vi "Hindbrain Main.vi"(8 "Boat Type":T1, 9 "XBee Serial Port":refnum<visa-resource-name>="LPT1", 11 "NotifierReff":T5) -> ()   [LabVIEW 2013]
doc: "Place to hold all the hindbrain code."
uses:
  Data/TypeDefs/Notifiers.ctl
  Data/TypeDefs/UTM Location.ctl
  Data/TypeDefs/Sail Set Suggestions.ctl
  Data/TypeDefs/Rudder Set Suggestions.ctl
  Data/TypeDefs/OverrideInformation.ctl
  Data/TypeDefs/OverrideMode.ctl
  Data/TypeDefs/MotorSetup.ctl
  Data/TypeDefs/DynamixelSetupInfo.ctl
  Data/TypeDefs/AirmarStatus.ctl
  Data/TypeDefs/HardwareOnline.ctl
  Data/TypeDefs/DynamixelCycleTracker.ctl
  Data/TypeDefs/RC Input Values.ctl
  Classes/Waypoint/Waypoint.lvclass
  Data/TypeDefs/BoatType.ctl
  <vilib>/myRIO/Common/Instrument Driver Framework/myRIO v1.0/UART/vis/myRIO v1.0 Close UART.vi
  <vilib>/myRIO/Common/Instrument Driver Framework/Utilities/vis/FPGA Ref Manager.vi
  <vilib>/myRIO/Common/Instrument Driver Framework/myRIO v1.0/myRIO v1.0 Reset FPGA.vi
  <vilib>/myRIO/Instrument Drivers/Utilities/Utilities.lvlib
  <instrlib>/Dynamixel Motor/Dynamixel Motor.lvlib
panel:
  in  "Tab Control":T2(tab)
  out "Write loop\ncounter":i32
  out "Commanded rudder value":T3 min=-0.95 max=0.95 scale=1.0..-1.0
  out "Commanded sail value":dbl
  out "Dynamixel\nPositions (deg)":dbl[](array[numeric])
  in  "Read actions per\nwrite action":i32=4
  out "Think Counter":i32
  out "Think Heartbeat":bool
  out "Sense Counter":i32
  out "Sense Heartbeat":bool
  out "Act Heartbeat":bool
  out "Read loop counter":i32
  out "Updated Dynamixel Cycles":T4
  in  "Motors Enabled":bool[](array[boolean])=[TRUE, TRUE, TRUE]
  out "Hemisphere Counter":i32
  out "Airmar Counter":i32
  out "Hemi Compass":dbl
  out "Airmar Compass":dbl
  out "String written to XBee":string
  out "String received from XBee":string
  out "UDP Time Out?":bool
  out "Battery Volts":dbl
  out "Replace? (<6?)":bool
  in  "Wind Speed":dbl
  out "XBee Sense/Act Counter":i32
  out "XBee Sense/Act Heartbeat":bool
  out "Camera Sense Counter":i32
  out "Camera Sense Heartbeat":bool
  out "Think Counter":i32
  out "Think Heartbeat":bool
  # "Timing"
  # "Timing"
  # "If you're getting no strings, do you have the right COM port?"
  # "Camera"
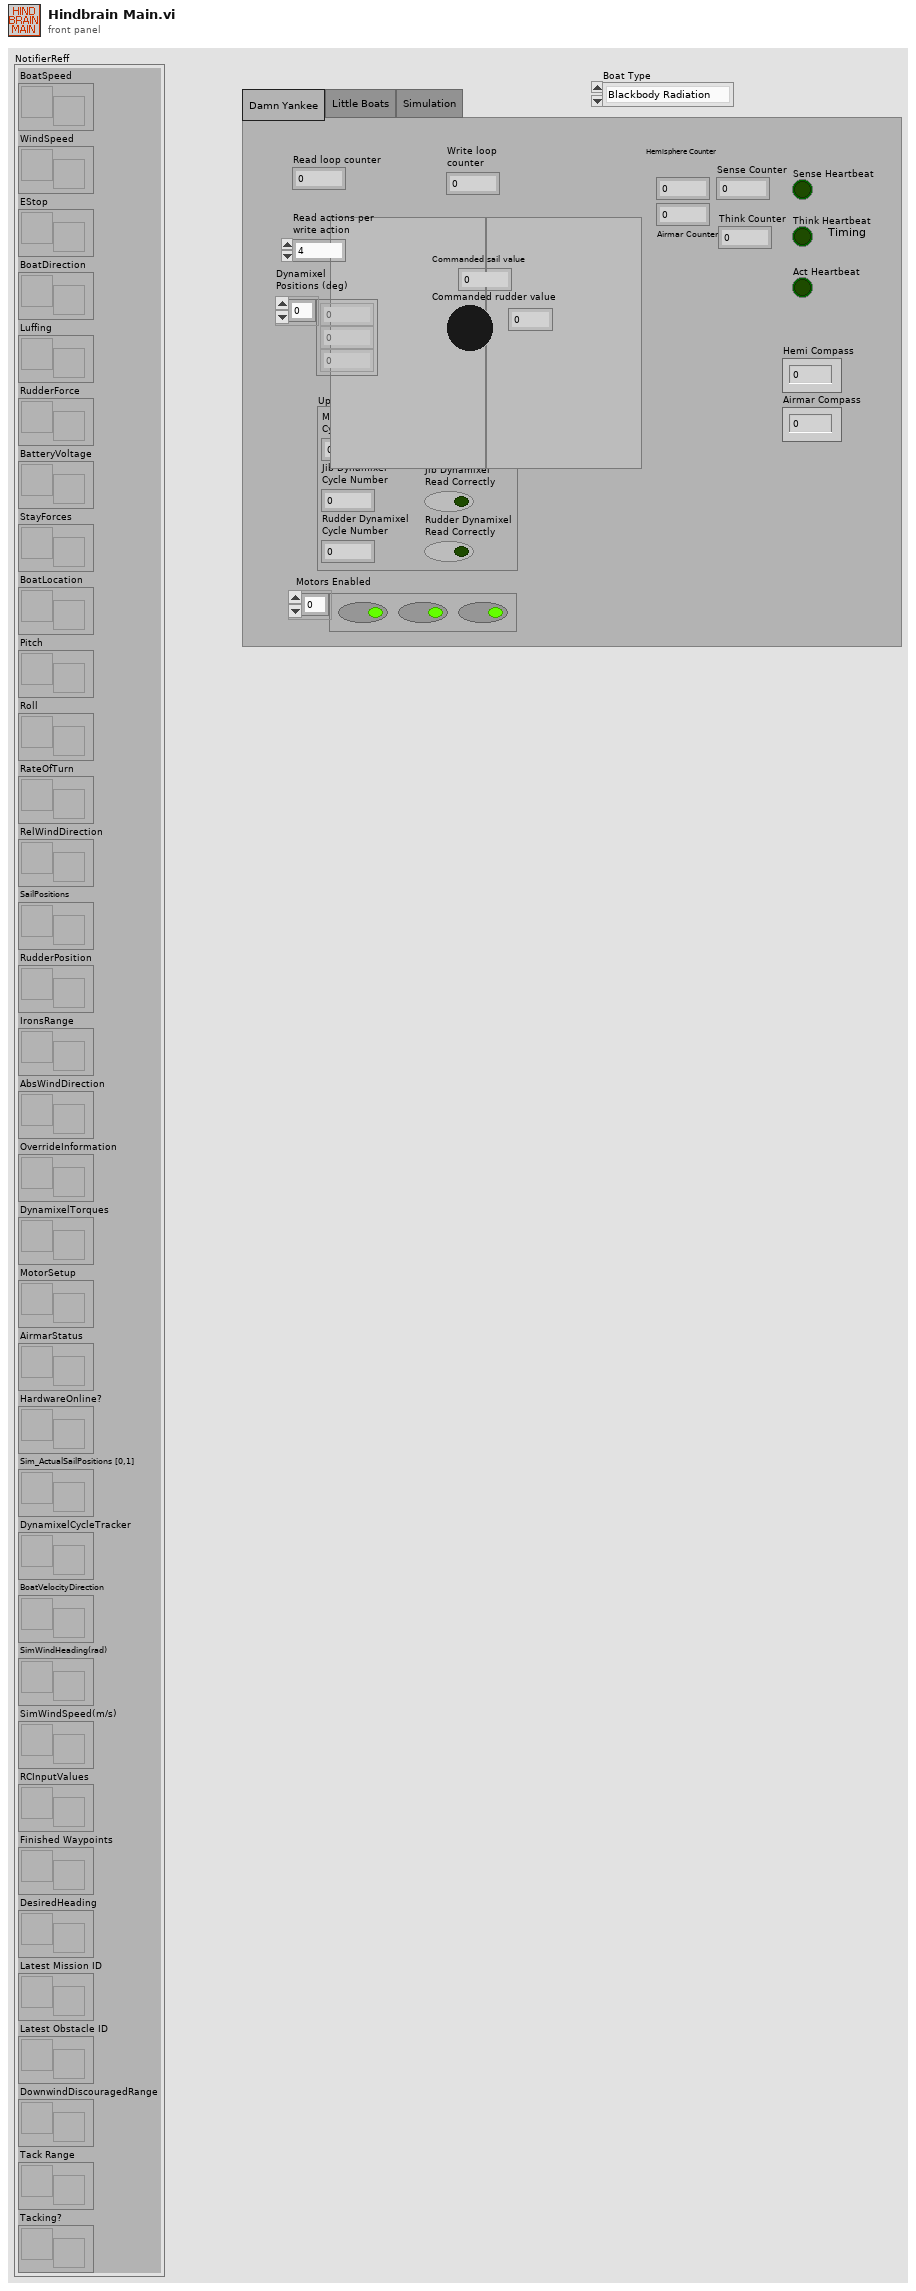
[diagram p1: front panel]
types:
  T1 = typedef "BoatType.ctl" = enum16{"Blackbody Radiation", "ReadLog", "Little boats", "Damn Yankee"}
  T2 = enum32{"Damn Yankee", "Little Boats", "Simulation"}
  T3 = typedef "Rudder Set Suggestions.ctl" = dbl
  T4 = typedef "DynamixelCycleTracker.ctl" = cluster{"Main Dynamixel\nCycle Number":i32, "Jib Dynamixel\nCycle Number":i32, "Rudder Dynamixel\nCycle Number":i32, "Main Dynamixel\nRead Correctly":bool, "Jib Dynamixel\nRead Correctly":bool, "Rudder Dynamixel\nRead Correctly":bool}
  T5 = typedef "Notifiers.ctl" = cluster{"BoatSpeed":refnum<notifier>, "WindSpeed":refnum<notifier>, "EStop":refnum<notifier>, "BoatDirection":refnum<notifier>, "Luffing":refnum<notifier>, "RudderForce":refnum<notifier>, "BatteryVoltage":refnum<notifier>, "StayForces":refnum<notifier>, "BoatLocation":refnum<notifier>, "Pitch":refnum<notifier>, "Roll":refnum<notifier>, "RateOfTurn":refnum<notifier>, "RelWindDirection":refnum<notifier>, "SailPositions":refnum<notifier>, "RudderPosition":refnum<notifier>, "IronsRange":refnum<notifier>, "AbsWindDirection":refnum<notifier>, "OverrideInformation":refnum<notifier>, "DynamixelTorques":refnum<notifier>, "MotorSetup":refnum<notifier>, "AirmarStatus":refnum<notifier>, "HardwareOnline?":refnum<notifier>, "Sim_ActualSailPositions [0,1]":refnum<notifier>, "DynamixelCycleTracker":refnum<notifier>, "BoatVelocityDirection":refnum<notifier>, "SimWindHeading(rad)":refnum<notifier>, "SimWindSpeed(m/s)":refnum<notifier>, "RCInputValues":refnum<notifier>, "Finished Waypoints":refnum<notifier>, "DesiredHeading":refnum<notifier>, "Latest Mission ID":refnum<notifier>, "Latest Obstacle ID":refnum<notifier>, "DownwindDiscouragedRange":refnum<notifier>, "Tack Range":refnum<notifier>, "Tacking?":refnum<notifier>}
  T6 = typedef "GPS-Compass Queue Cluster.ctl" = cluster{"BoatLocation Queue":refnum<queue>, "BoatDirection Queue":refnum<queue>, "BoatSpeed Queue":refnum<queue>, "RateOfTurn Queue":refnum<queue>, "Pitch Queue":refnum<queue>, "Roll Queue":refnum<queue>, "BoatVelocityDirection Queue ":refnum<queue>}
  T7 = typedef "WindData Queue Cluster.ctl" = cluster{"RelWindDirection Queue":refnum<queue>, "WindSpeed Queue":refnum<queue>, "AbsWindDirection Queue":refnum<queue>}
  T8 = cluster{"Shroud Queue":refnum<queue>, "Battery Voltage Queue":refnum<queue>, "Accelerometer Queue":refnum<queue>, "AirmarGPS-Compass Queue Cluster":T6, "Hemisphere Queue Cluster":T6, "Airmar Wind Queue Cluster":T7, "Wind Vane Queue Cluster":T7, "Little Boat Queues":cluster{"Heading Queue":refnum<queue>, "Location Queue":refnum<queue>, "Wind Speed Queue":refnum<queue>, "Tilt Queue":refnum<queue>, "Wind Direction Queue":refnum<queue>}, "DynamixelTorque Queue":refnum<queue>, "DynamixelPosition Queue":refnum<queue>}
  T9 = typedef "MotorSetup.ctl" = cluster{"Main Dynamixel Set Data":T10, "Rudder Dynamixel Set Data":T10, "Jib Dynamixel Set Data":T10}
  T10 = typedef "DynamixelSetupInfo.ctl" = cluster{"Lower Winch Bound (deg)":dbl, "Upper Winch Bound (deg)":dbl}
  T11 = typedef "DamnYankeeIOPorts.ctl" = cluster{"Airmar VISA Resource":refnum<visa-resource-name>, "Hemisphere VISA Resource":refnum<visa-resource-name>, "Dynamixel VISA Resource":refnum<visa-resource-name>, "Airmar Error":errorcluster, "Hemisphere Error":errorcluster, "Dynamixel Error":errorcluster, "FPGA Error":errorcluster, "FPGA VI Reference Out":refnum<k20>, "Motors IDs Found":u8[]}
  T12 = cluster{"Heading Queue":refnum<queue>, "Location Queue":refnum<queue>, "Wind Speed Queue":refnum<queue>, "Tilt Queue":refnum<queue>, "Wind Direction Queue":refnum<queue>}
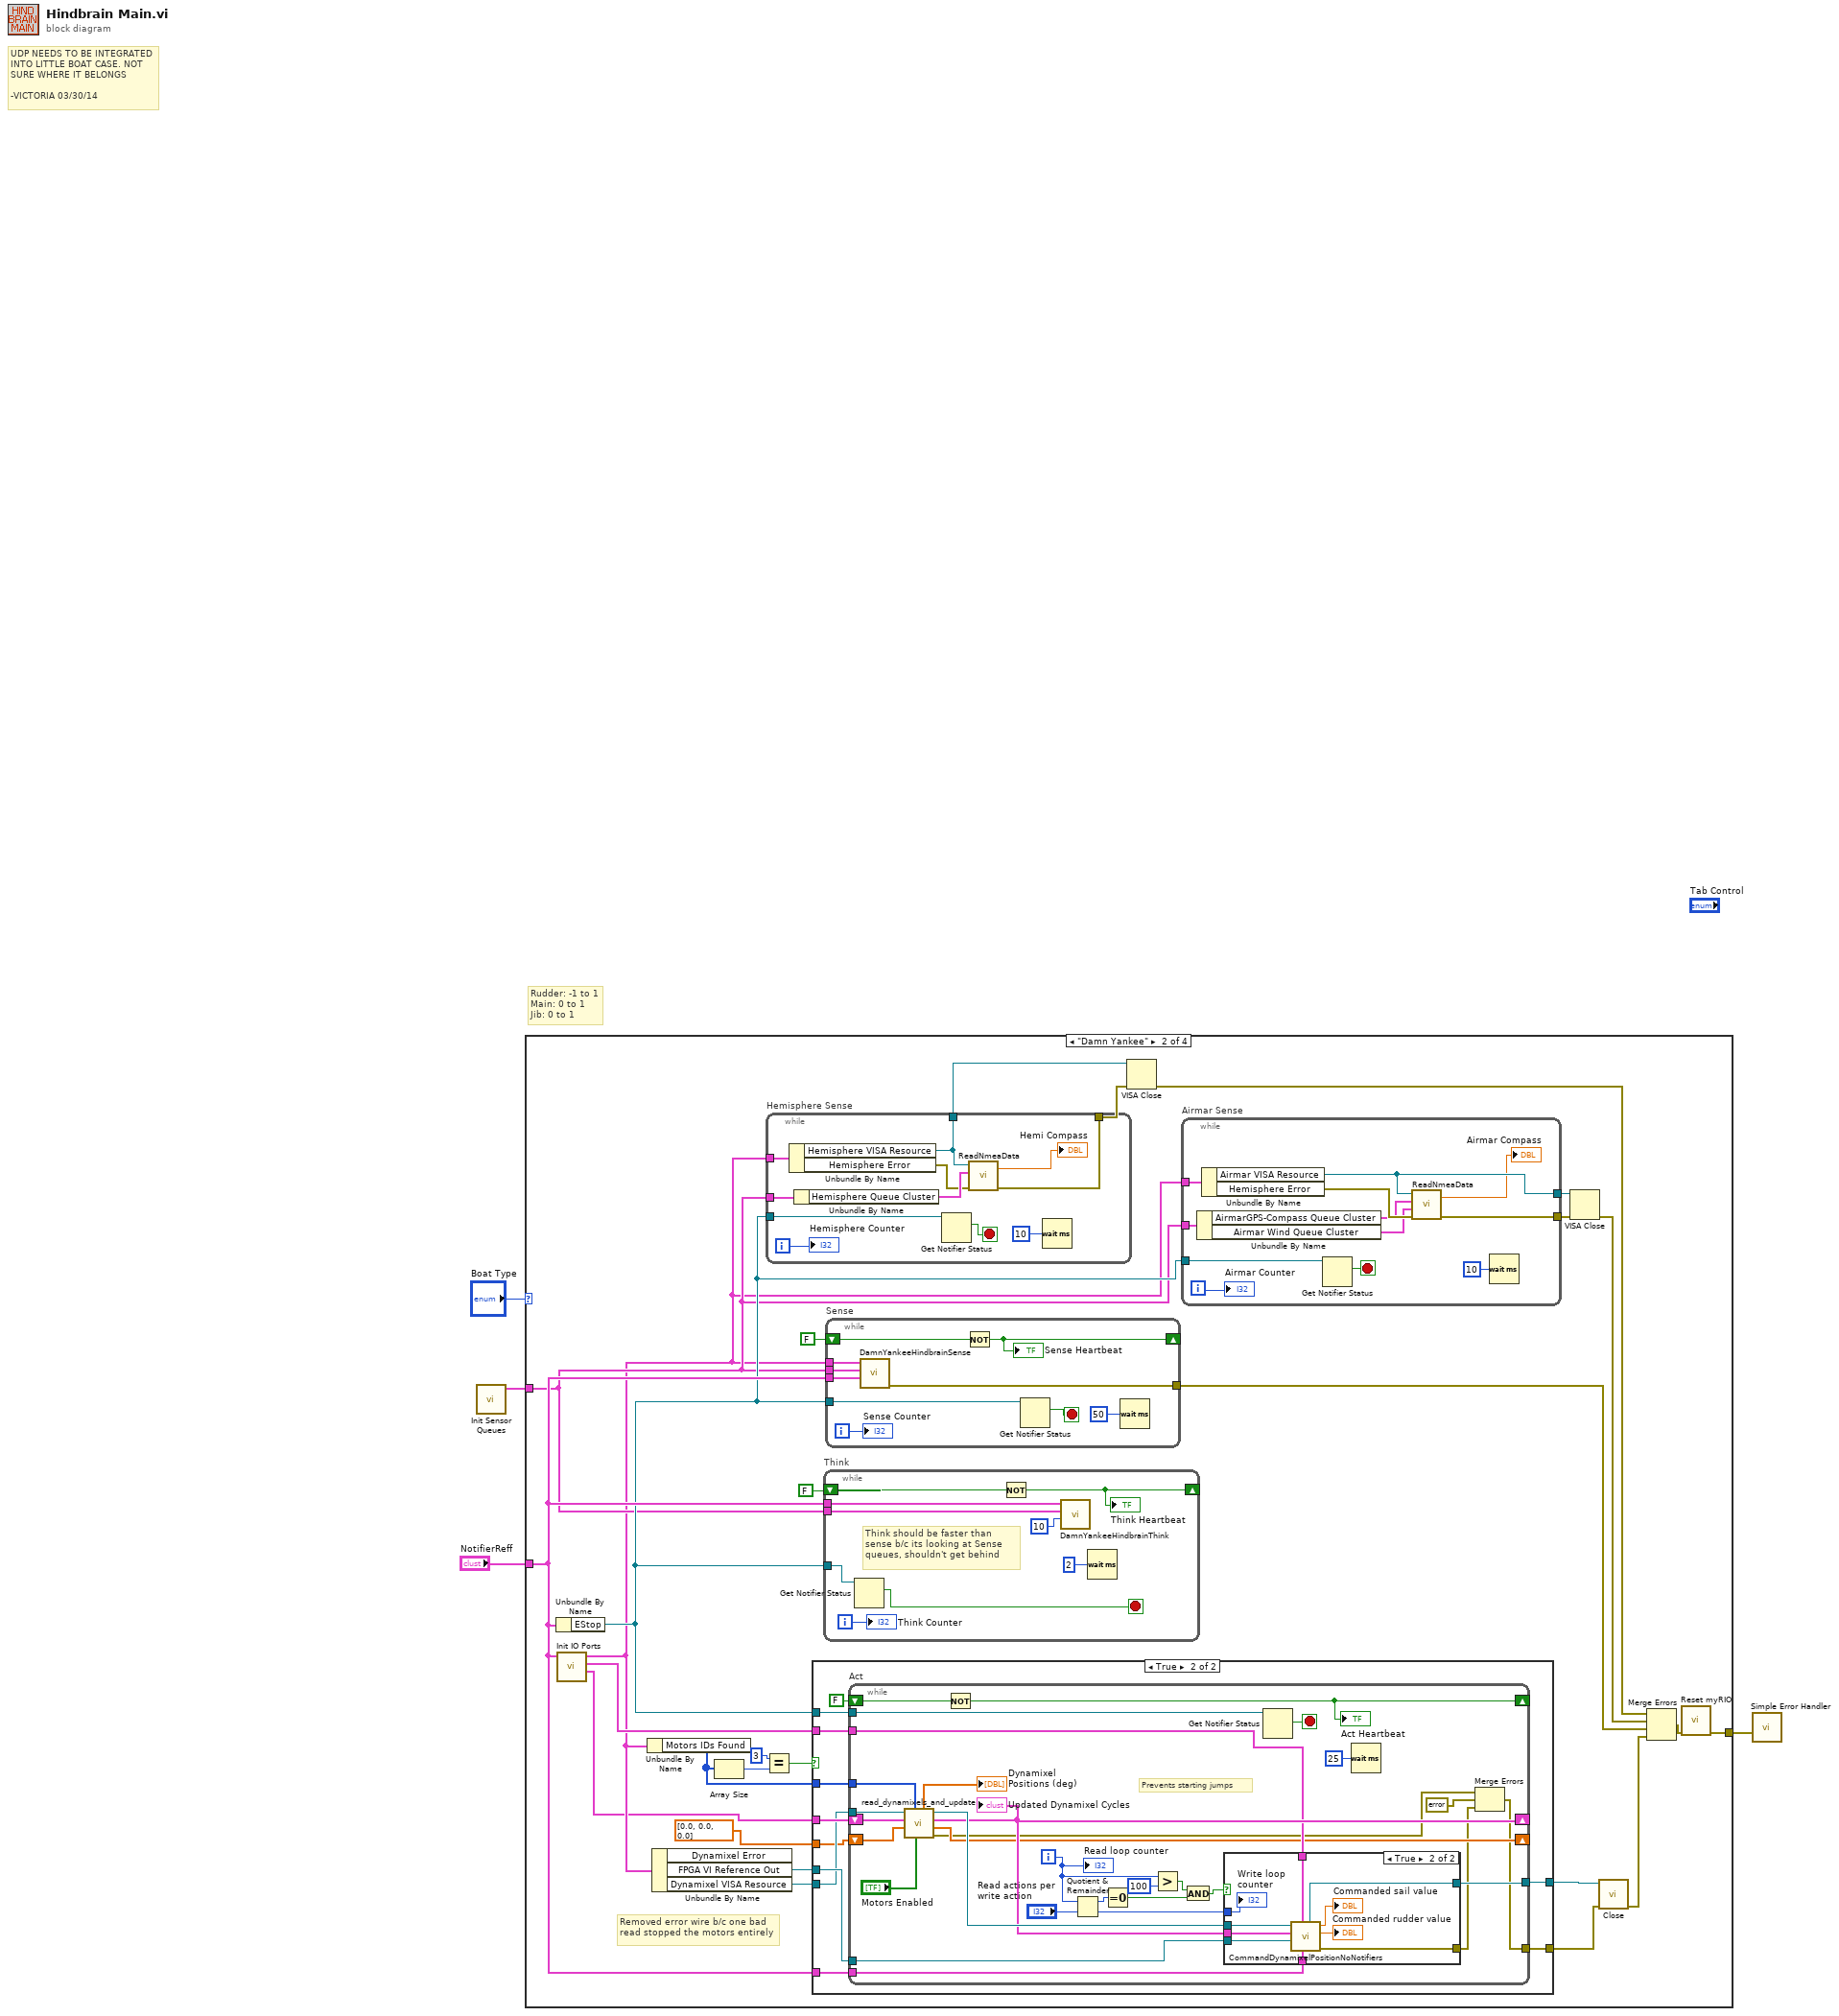
[diagram p0: block diagram]
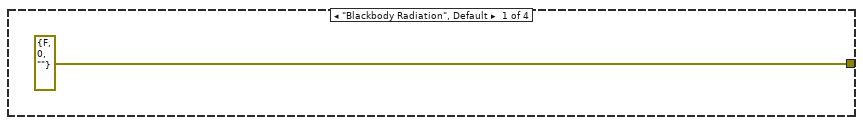
[diagram p2: hidden frame]
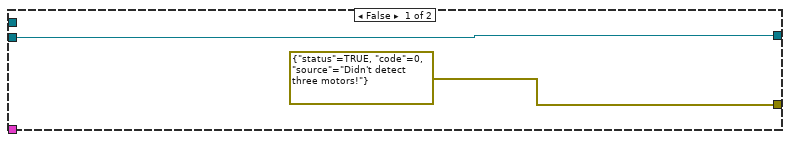
[diagram p3: hidden frame]
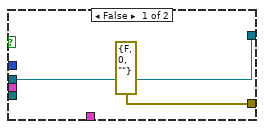
[diagram p4: hidden frame]
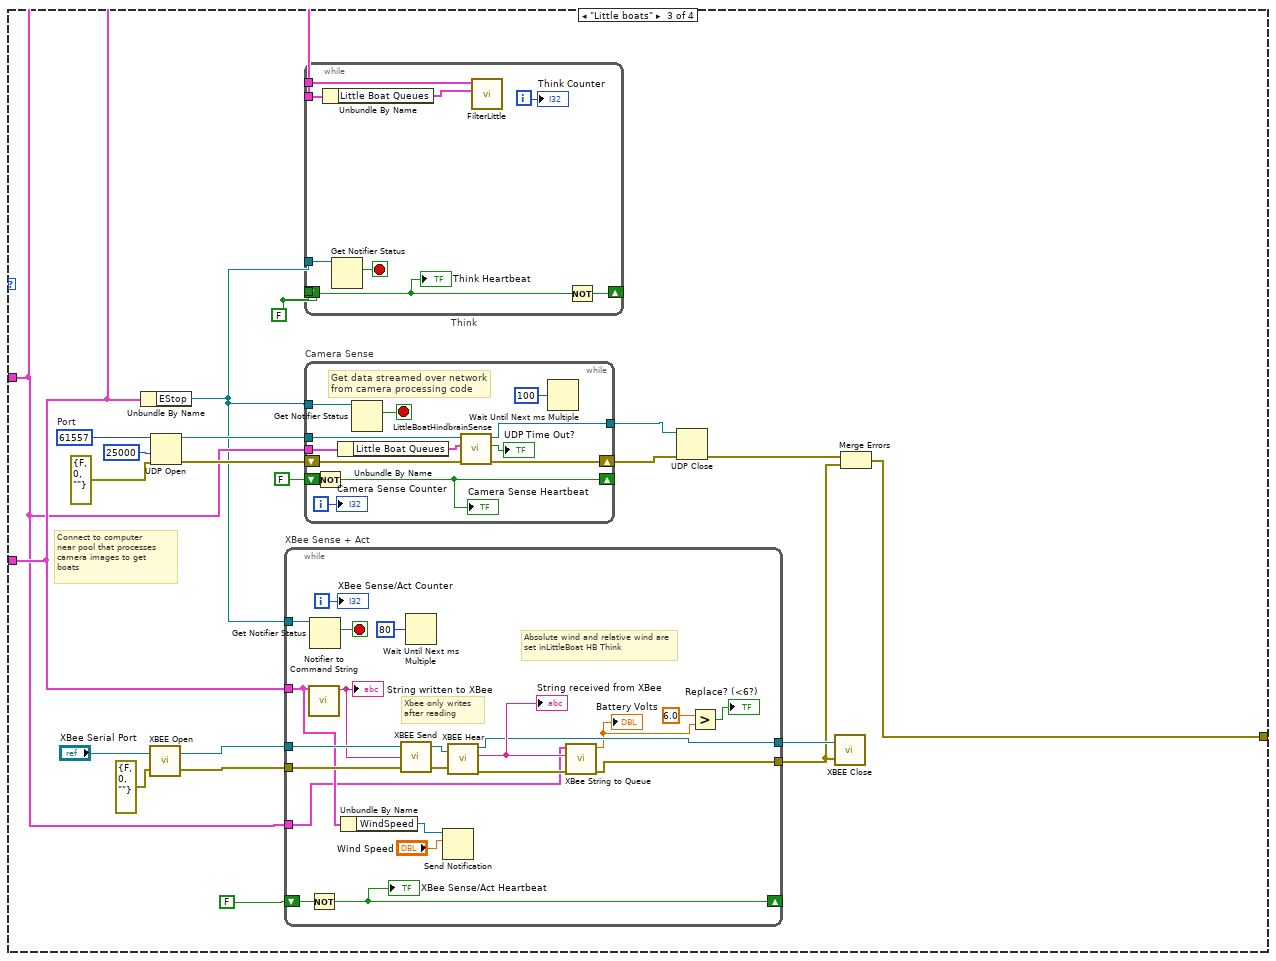
[diagram p5: hidden frame]
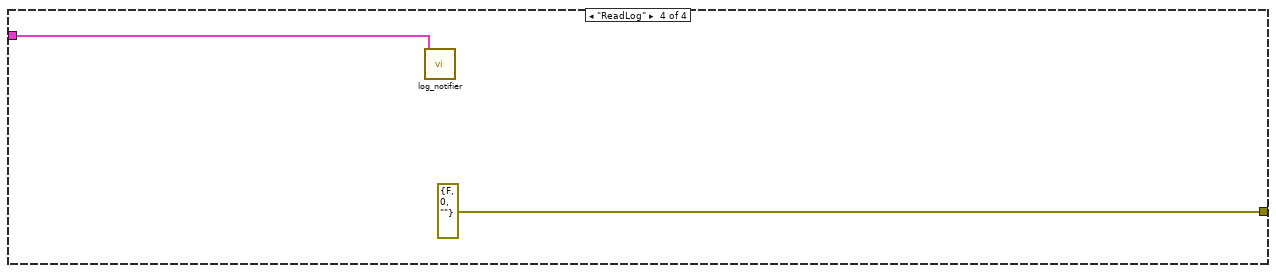
[diagram p6: hidden frame]
diagram:
  # "Rudder: -1 to 1\nMain: 0 to 1 \nJib: 0 to 1"
  # "UDP NEEDS TO BE INTEGRATED\nINTO LITTLE BOAT CASE. NOT \nSURE WHERE IT BELONGS\n\n-VICTORIA 03/30/14"
  n1 = call "Init Sensor Queues.vi"() -> ("output cluster"=w4:T8)  [unwired: 11 in]
  n2 = case shown="\"Damn Yankee\"" "Boat Type" {
    tunnel: w4 -> [_ w15 w139 _]
    tunnel: "NotifierReff" -> [_ w18 w143 w194]
    tunnel: [errorcluster {"status"=FALSE, "code"=0, "source"=""} ("error IO") w31 w150 errorcluster {"status"=FALSE, "code"=0, "source"=""} ("error IO")] -> w3
    frame "Blackbody Radiation", Default {
    }
    frame "Damn Yankee" {
      # "Removed error wire b/c one bad read stopped the motors entirely"
      n3 = Unbundle By Name(w18) -> ("EStop"=w16:refnum<notifier>)
      n4 = call "Init IO Ports.vi"("NotifierReff"=w18) -> ("Dynamixel Cycles"=w6:T4, "Dynamixel Bounds Out"=w23:T9, "IO Port Cluster"=w14:T11)  [unwired: 8 in]
      n5 = Unbundle By Name(w14) -> ("Motors IDs Found"=w24:u8[])
      n6 = Unbundle By Name(w14) -> ("FPGA VI Reference Out"=w25:refnum<k20>, "Dynamixel VISA Resource"=w22:refnum<visa-resource-name>)  [unwired: 1 out]
      n7 = Array Size(array=w24) -> (size(s)=w28:i32)
      n8 = Equal?(x=3, y=w28) -> (x = y?=w27:bool)
      n9 = while "Hemisphere Sense" {
        tunnel: w14 -> [w55]
        tunnel: w15 -> [w54]
        tunnel: w16 -> [w50]
        tunnel: [w48] -> w13
        tunnel: [w47] -> w12
        i -> [w51]
        stop <- w49 stop-if-true
        n10 = Unbundle By Name(w55) -> ("Hemisphere VISA Resource"=w48:refnum<visa-resource-name>, "Hemisphere Error"=w52:errorcluster)
        n11 = Unbundle By Name(w54) -> ("Hemisphere Queue Cluster"=w53:T6)
        n12 = Get Notifier Status(notifier=w50) -> (current notification=w49:bool)  [unwired: 1 in, 4 out]
        n13 = call "ReadNmeaData.vi"("error in"=w52, "GPS-Compass Queue Cluster"=w53, "Serial Port"=w48) -> ("error out"=w47:errorcluster, "Boat Direction 2"=→"Hemi Compass":dbl)  [unwired: 2 in, 5 out]
        n14 = Wait (ms)(milliseconds to wait=u32 10) -> ()  [unwired: 1 out]
        "Hemisphere Counter" <- w51
      }
      n15 = case shown="True" w27 {
        tunnel: [errorcluster {"status"=TRUE, "code"=0, "source"="Didn't detect three motors!"} ("error out") w58] -> w20
        tunnel: w16 -> [_ w67]
        tunnel: w23 -> [_ w66]
        tunnel: w6 -> [_ w65]
        tunnel: [w56 w64] -> w21
        tunnel: w25 -> [_ w63]
        tunnel: w24 -> [_ w62]
        tunnel: w22 -> [w56 w61]
        tunnel: w18 -> [_ w60]
        tunnel: dbl[] [0.0, 0.0, 0.0] -> [_ w59]
        frame False {
        }
        frame True {
          n16 = while "Act" {
            tunnel: w66 -> [w85]
            tunnel: w67 -> [w97]
            shift-right: [w96] -> _
            shift-left: FALSE -> [w95]
            shift-right: [w86] -> _
            shift-left: w65 -> [w87]
            tunnel: [w84] -> w64
            shift-right: [w83] -> _
            shift-left: w59 -> [w82]
            tunnel: w63 -> [w79]
            tunnel: w62 -> [w78]
            tunnel: w61 -> [w77]
            tunnel: w60 -> [w76]
            tunnel: [w74] -> w58
            i -> [w71]
            stop <- w98 stop-if-true
            # "Prevents starting jumps"
            n17 = call "read_dynamixels_and_update.vi"("Motors Enabled"="Motors Enabled", "Motors IDs Found"=w78, "Last read positions"=w82, "Dynamixel Cycle Constant"=w87, "VISA Refnum in"=w77) -> ("error out"=w81:errorcluster[], "Latest read positions (dyn)"=w83:dbl[], "Updated Dynamixle Cycles"=w86:T4, "VISA Refnum out"=w92:refnum<visa-resource-name>, "Dynamixel\nPositions (deg)"=→"Dynamixel\nPositions (deg)":dbl[])  [unwired: 2 in]
            "Updated Dynamixel Cycles" <- w86
            n18 = Not(x=w95) -> (.not. x?=w96:bool)
            "Act Heartbeat" <- w96
            n19 = Quotient & Remainder(x=w71, y="Read actions per\nwrite action") -> (x-y*floor(x/y)=w90:i32, floor(x/y)=w89:i32)
            n20 = Equal To 0?(x=w90) -> (x = 0?=w72:bool)
            n21 = Greater?(x=w71, y=100) -> (0:w70:bool)
            n22 = And(x=w70, y=w72) -> (x .and. y?=w73:bool)
            n23 = case shown="True" w73 {
              tunnel: w79 -> [_ w110]
              tunnel: w85 -> [_ w102]
              tunnel: w92 -> [w100 w109]
              tunnel: w86 -> [_ w108]
              tunnel: [errorcluster {"status"=FALSE, "code"=0, "source"=""} ("Error out") w105] -> w75
              tunnel: [w100 w104] -> w84
              tunnel: w89 -> [_ w103]
              tunnel: w76 -> [_ w101]
              frame False {
              }
              frame True {
                n24 = call "CommandDynamixelPositionNoNotifiers.vi"("NotifierReff"=w101, "Dynamixel Bounds"=w102, "FPGA VI Reference In"=w110, "Dynamixel Cycles"=w108, "VISA resource name"=w109) -> ("Error out"=w105:errorcluster, "Commanded rudder value"=→"Commanded rudder value":T3, "Debug sail value"=→"Commanded sail value":dbl, "VISA resource name OUT"=w104:refnum<visa-resource-name>)  [unwired: 3 in]
                "Write loop\ncounter" <- w103
              }
            }
            n25 = Get Notifier Status(notifier=w97) -> (current notification=w98:bool)  [unwired: 1 in, 4 out]
            n26 = Wait (ms)(milliseconds to wait=u32 25) -> ()  [unwired: 1 out]
            n27 = Merge Errors(w81, errorcluster {"status"=FALSE, "code"=0, "source"=""} ("error IO"), w75) -> (w74:errorcluster)
            "Read loop counter" <- w71
          }
        }
      }
      n28 = while "Think" {
        tunnel: w16 -> [w119]
        tunnel: w15 -> [w113]
        tunnel: w18 -> [w117]
        shift-right: [w114] -> _
        shift-left: FALSE -> [w115]
        i -> [w116]
        stop <- w118 stop-if-true
        # "Think should be faster than sense b/c its looking at Sense queues, shouldn't get behind"
        n29 = Get Notifier Status(notifier=w119) -> (current notification=w118:bool)  [unwired: 1 in, 4 out]
        n30 = Not(x=w115) -> (.not. x?=w114:bool)
        "Think Heartbeat" <- w114
        n31 = call "DamnYankeeHindbrainThink.vi"("Queue timeout (ms)"=10, "Data queue cluster"=w113, "Notifier References"=w117) -> ()  [unwired: 9 in]
        n32 = Wait (ms)(milliseconds to wait=u32 2) -> ()  [unwired: 1 out]
        "Think Counter" <- w116
      }
      n33 = while "Sense" {
        tunnel: w14 -> [w121]
        tunnel: w18 -> [w129]
        tunnel: w15 -> [w125]
        tunnel: [w128] -> w7
        tunnel: w16 -> [w127]
        shift-right: [w122] -> _
        shift-left: FALSE -> [w123]
        i -> [w124]
        stop <- w126 stop-if-true
        n34 = call "DamnYankeeHindbrainSense.vi"("Notifier References"=w129, "Data Queue clusters"=w125, "IO Cluster"=w121) -> ("error out"=w128:errorcluster)  [unwired: 8 in]
        n35 = Not(x=w123) -> (.not. x?=w122:bool)
        "Sense Heartbeat" <- w122
        n36 = Get Notifier Status(notifier=w127) -> (current notification=w126:bool)  [unwired: 1 in, 4 out]
        n37 = Wait (ms)(milliseconds to wait=u32 50) -> ()  [unwired: 1 out]
        "Sense Counter" <- w124
      }
      n38 = VISA Close(VISA resource name=w13, error in (no error)=w12) -> (error out=w10:errorcluster)
      n39 = while "Airmar Sense" {
        tunnel: w14 -> [w44]
        tunnel: w15 -> [w43]
        tunnel: w16 -> [w41]
        tunnel: [w39] -> w11
        tunnel: [w34] -> w8
        i -> [w42]
        stop <- w40 stop-if-true
        n40 = Unbundle By Name(w43) -> ("AirmarGPS-Compass Queue Cluster"=w36:T6, "Airmar Wind Queue Cluster"=w37:T7)
        n41 = Unbundle By Name(w44) -> ("Airmar VISA Resource"=w34:refnum<visa-resource-name>, "Hemisphere Error"=w38:errorcluster)
        n42 = Get Notifier Status(notifier=w41) -> (current notification=w40:bool)  [unwired: 1 in, 4 out]
        n43 = call "ReadNmeaData.vi"("error in"=w38, "Airmar Wind Queue Cluster"=w37, "GPS-Compass Queue Cluster"=w36, "Serial Port"=w34) -> ("error out"=w39:errorcluster, "Boat Direction 2"=→"Airmar Compass":dbl)  [unwired: 1 in, 5 out]
        n44 = Wait (ms)(milliseconds to wait=u32 10) -> ()  [unwired: 1 out]
        "Airmar Counter" <- w42
      }
      n45 = VISA Close(VISA resource name=w8, error in (no error)=w11) -> (error out=w9:errorcluster)
      n46 = call <instrlib>:"Close.vi"("error in (no error)"=w20, "VISA resource name"=w21) -> ("error out"=w19:errorcluster)  [unwired: 9 in]
      n47 = Merge Errors "Merge Errors"(w10, w9, w7, w19) -> (w32:errorcluster)
      n48 = call <vilib>:"Reset myRIO.vi"("error in (no error)"=w32) -> ("error out"=w31:errorcluster)  [unwired: 10 in]
    }
    frame "Little boats" {
      w130 = FALSE
      w148 = u16 61557  # Port
      # "Connect to computer\nnear pool that processes\ncamera images to get\nboats"
      n49 = Unbundle By Name(w143) -> ("EStop"=w133:refnum<notifier>)
      n50 = call "XBEE Open.vi"("error in"=errorcluster {"status"=FALSE, "code"=0, "source"=""}, "VISA resource name"="XBee Serial Port") -> ("error out"=w142:errorcluster, "VISA resource name out"=w144:refnum<visa-resource-name>)
      n51 = UDP Open(8:errorcluster {"status"=FALSE, "code"=0, "source"=""} ("error in (no error)"), 9:25000 ("timeout ms (25000)"), 11:w148) -> (port=w141:refnum<k16>, 0:w140:errorcluster)  [unwired: 2 in, 1 out]
      n52 = while "XBee Sense + Act" {
        tunnel: w144 -> [w184]
        tunnel: w143 -> [w170]
        tunnel: w133 -> [w185]
        tunnel: w139 -> [w165]
        tunnel: [w175] -> w138
        tunnel: w142 -> [w183]
        tunnel: [w174] -> w137
        shift-right: [w167] -> _
        shift-left: FALSE -> [w168]
        i -> [w166]
        stop <- w179 stop-if-true
        # "Absolute wind and relative wind are set inLittleBoat HB Think"
        # "Xbee only writes\nafter reading"
        n53 = call "Notifier to Command String.vi"("NotifierReff"=w170) -> ("String"=w182:string)  [unwired: 10 in]
        "String written to XBee" <- w182
        n54 = Not(x=w168) -> (.not. x?=w167:bool)
        "XBee Sense/Act Heartbeat" <- w167
        n55 = Get Notifier Status(notifier=w185) -> (current notification=w179:bool)  [unwired: 1 in, 4 out]
        n56 = Unbundle By Name(w170) -> ("WindSpeed"=w169:refnum<notifier>)
        n57 = call "XBEE Send.vi"("error in (no error)"=w183, "String"=w182, "VISA resource name"=w184) -> ("error out"=w180:errorcluster, "VISA resource name out"=w181:refnum<visa-resource-name>)  [unwired: 1 out]
        n58 = Wait Until Next ms Multiple(millisecond multiple=u32 80) -> ()  [unwired: 1 out]
        n59 = Send Notification(notification="Wind Speed", notifier=w169) -> ()  [unwired: 1 in, 2 out]
        n60 = call "XBEE Hear.vi"("VISA resource name"=w181, "error in (no error)"=w180) -> ("VISA resource name out"=w175:refnum<visa-resource-name>, "String Received"=w178:string, "error out"=w177:errorcluster)  [unwired: 1 out]
        "String received from XBee" <- w178
        n61 = call "XBee String to Queue.vi"("error in (no error)"=w177, "String Received"=w178, "Queue cluster"=w165) -> ("error out"=w174:errorcluster, "Battery Volts"=w173:dbl)  [unwired: 7 in]
        "Battery Volts" <- w173
        n62 = Greater?(x=6.0, y=w173) -> (0:→"Replace? (<6?)":bool)
        "XBee Sense/Act Counter" <- w166
      }
      n63 = while "Think" {
        tunnel: w133 -> [w193]
        tunnel: w139 -> [w191]
        tunnel: w143 -> [w189]
        shift-right: [w187] -> _
        shift-left: w130 -> [w186]
        tunnel: w130 -> [_]
        i -> [w188]
        stop <- w192 stop-if-true
        n64 = Unbundle By Name(w191) -> ("Little Boat Queues"=w190:T12)
        n65 = Get Notifier Status(notifier=w193) -> (current notification=w192:bool)  [unwired: 1 in, 4 out]
        n66 = call "FilterLittle.vi"("Little Boat Queues"=w190, "NotifierReff"=w189) -> ()  [unwired: 10 in]
        n67 = Not(x=w186) -> (.not. x?=w187:bool)
        "Think Counter" <- w188
        "Think Heartbeat" <- w186
      }
      n68 = while "Camera Sense" {
        tunnel: w141 -> [w162]
        tunnel: w139 -> [w161]
        tunnel: [w159] -> w136
        tunnel: w133 -> [w156]
        shift-right: [w158] -> w135
        shift-left: w140 -> [w163]
        shift-right: [w151] -> _
        shift-left: FALSE -> [w152]
        i -> [w153]
        stop <- w155 stop-if-true
        # "Get data streamed over network from camera processing code"
        n69 = Not(x=w152) -> (.not. x?=w151:bool)
        "Camera Sense Heartbeat" <- w151
        n70 = Unbundle By Name(w161) -> ("Little Boat Queues"=w160:T12)
        n71 = Get Notifier Status(notifier=w156) -> (current notification=w155:bool)  [unwired: 1 in, 4 out]
        n72 = call "LittleBoatHindbrainSense.vi"("error in (no error)"=w163, "Little Boat Queues"=w160, "connection ID"=w162) -> ("error out"=w158:errorcluster, "UDP Time Out?"=→"UDP Time Out?":bool, "connection ID out"=w159:refnum<k16>)  [unwired: 6 in]
        n73 = Wait Until Next ms Multiple(millisecond multiple=u32 100) -> ()  [unwired: 1 out]
        "Camera Sense Counter" <- w153
      }
      n74 = UDP Close(connection ID=w136, 8:w135) -> (error out=w134:errorcluster)  [unwired: 1 out]
      n75 = call "XBEE Close.vi"("error in (no error)"=w137, "VISA resource name"=w138) -> ()
      n76 = Merge Errors "Merge Errors"(w134, w137) -> (w150:errorcluster)
    }
    frame "ReadLog" {
      n77 = call "log_notifier.vi"("NotifierReferences"=w194) -> ()  [unwired: 11 in]
    }
  }
  n78 = call <vilib>:"Simple Error Handler.vi"("error in (no error)"=w3) -> ()  [unwired: 4 in, 5 out]
